vi "Test.vi"() -> ()   [LabVIEW 2022 SP3, in "EMKO.lvlib" / "ESM-xx50.lvclass"]
uses:
  ESM-xx50.lvclass
  ESM-xx50.lvclass/ESM-xx50.ctl
panel:
  out "Process Variable":u16
  out "Process SV":u16
  out "error out":errorcluster
  in  "Serial Port":string="COM7"
  in  "baud rate (9600)":u32=19200
  in  "Slave ID":u8=1
  in  "parity (Even)":u16(ring)=2 items=["None", "Odd", "Even"]
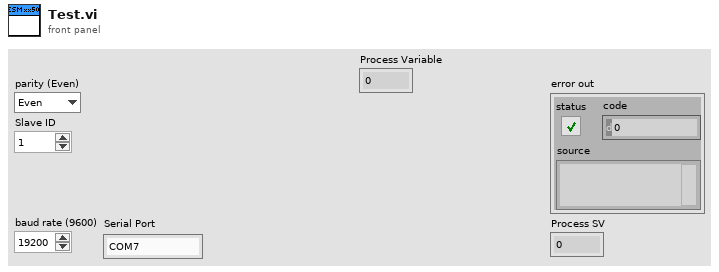
[diagram p1: front panel]
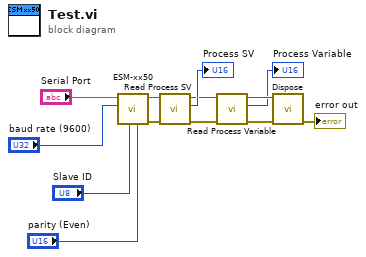
[diagram p0: block diagram]
diagram:
  n1 = call "ESM-xx50.vi"("parity"="parity (Even)", "Slave ID"="Slave ID", "baud rate (9600)"="baud rate (9600)", "Serial Port"="Serial Port") -> ("error out"=w8:errorcluster, "EMKO Out"=w9:refnum<class "ESM-xx50.lvclass">)  [unwired: 6 in]
  n2 = call-dynamic "Read Process SV.vi"("error in (no error)"=w8, "EMKO in"=w9) -> ("error out"=w2:errorcluster, "Process SV"=→"Process SV":u16, "EMKO out"=w5:refnum<class "ESM-xx50.lvclass">)  [unwired: 7 in]
  n3 = call-dynamic "Read Process Variable.vi"("error in (no error)"=w2, "EMKO in"=w5) -> ("error out"=w3:errorcluster, "Process Variable"=→"Process Variable":u16, "EMKO out"=w4:refnum<class "ESM-xx50.lvclass">)  [unwired: 7 in]
  n4 = call "Dispose.vi"("error in (no error)"=w3, "EMKO"=w4) -> ("error out"=→"error out":errorcluster)  [unwired: 9 in]
